vi "UI V7.1.1.vi"() -> ()   [LabVIEW 2017]
uses:
  <vilib>/Instr/_visa.llb/VISA Configure Serial Port (Instr).vi
  <vilib>/addons/Biomedical/Biosignal Measurements/Biosignal Preprocessing/Biosignal Rate Extractor (Waveform).vi
  <vilib>/addons/Biomedical/NI_BMTK_Measurements.lvlib
panel:
  out "?":bool
  out "?":bool
  out "CH1 PULSE Counter PM":u8
  out "CH2 PULSE Counter PM":i32
  out "CH1 PM":u8
  out "CH2 PM":dbl format="%#.6g"
  out "CH2":waveform(dbl)(graph)
  in  "stop":bool
  out "CH1":waveform(dbl)(graph)
  in  "Arduino Port":refnum<visa-resource-name>
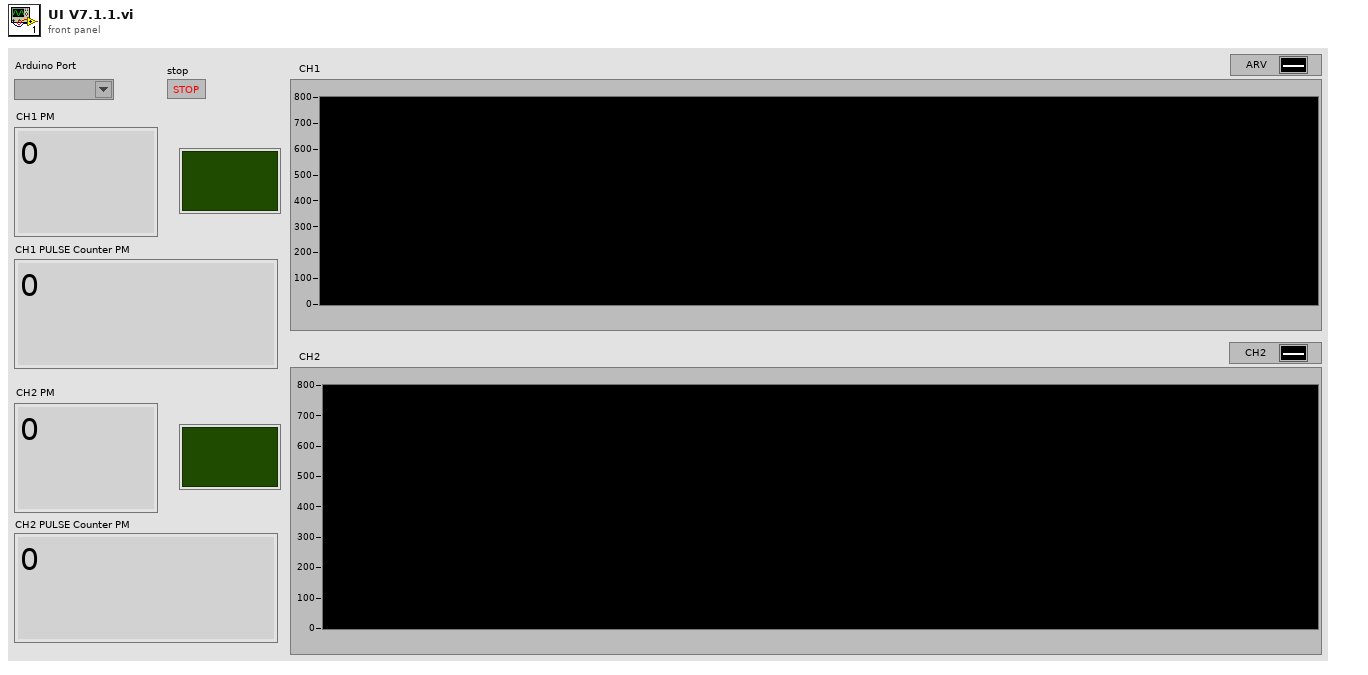
[diagram p1: front panel]
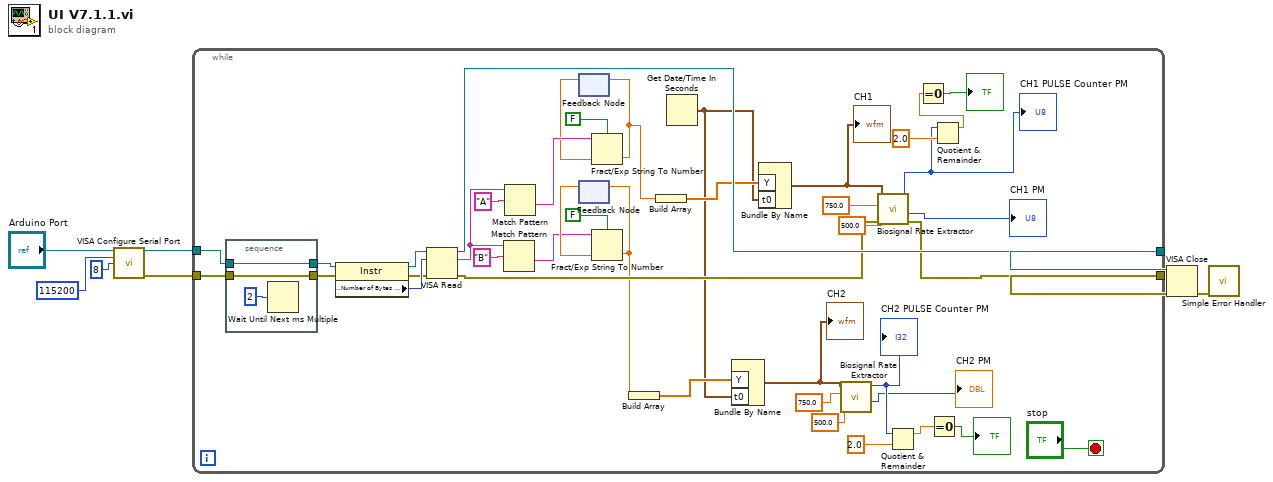
[diagram p0: block diagram]
diagram:
  n1 = call-poly "VISA Configure Serial Port"("VISA resource name"="Arduino Port", "baud rate (9600)"=u32 115200, "data bits (8)"=u16 8) -> ("VISA resource name out"=w5:refnum<visa-resource-name>, "error out"=w4:errorcluster)  [unwired: 11 in]
  n2 = while {
    tunnel: w5 -> [w49]
    tunnel: w4 -> [w47]
    tunnel: [w34] -> w3
    tunnel: [w28] -> w2
    stop <- "stop" stop-if-true
    n3 = stacked-sequence {
      tunnel: w49 -> [w52]
      tunnel: [w52] -> w48
      tunnel: w47 -> [w51]
      tunnel: [w51] -> w46
      frame #0 {
        n4 = Wait Until Next ms Multiple(millisecond multiple=u32 2) -> ()  [unwired: 1 out]
      }
    }
    n5 = property class="Instr"(reference=w48, error in=w46) -> (reference out=w45:refnum<visa-resource-name>, error out=w43:errorcluster, "Serial Settings:Number of Bytes at Serial Port"=w44:u32)
    n6 = VISA Read(VISA resource name=w45, byte count=w44, error in (no error)=w43) -> (VISA resource name out=w34:refnum<visa-resource-name>, read buffer=w33:string, error out=w29:errorcluster)  [unwired: 1 out]
    n7 = Match Pattern(string=w33, regular expression="B") -> (after substring=w32:string)  [unwired: 1 in, 3 out]
    n8 = Match Pattern(string=w33, regular expression="A") -> (after substring=w39:string)  [unwired: 1 in, 3 out]
    n9 = feedback #1() -> (w36:dbl)  [unwired: 1 in]
    n10 = feedback #2() -> (w35:dbl)  [unwired: 1 in]
    n11 = Fract/Exp String To Number(use system decimal point (T)=FALSE, string=w39, default (0 dbl)=w36) -> (number=w31:dbl)  [unwired: 1 in, 1 out]
    n12 = feedback-in #1(w31) -> ()
    n13 = Fract/Exp String To Number(use system decimal point (T)=FALSE, string=w32, default (0 dbl)=w35) -> (number=w21:dbl)  [unwired: 1 in, 1 out]
    n14 = feedback-in #2(w21) -> ()
    n15 = Build Array(w21) -> (w22:dbl[])
    n16 = Build Array(w31) -> (w30:dbl[])
    n17 = Get Date/Time In Seconds() -> (seconds since 1Jan1904=w13:timestamp)
    n18 = Bundle By Name("Y"=w22, "t0"=w13) -> (w23:waveform(dbl))  [unwired: 1 in]
    "CH2" <- w23
    n19 = Bundle By Name("Y"=w30, "t0"=w13) -> (w11:waveform(dbl))  [unwired: 1 in]
    "CH1" <- w11
    n20 = call-poly <vilib>:"Biosignal Rate Extractor.vi"("low threshold"=500.0, "high threshold"=750.0, "biosignal"=w23) -> ("number of cycles per minuets"=→"CH2 PM":i32, "number of cycles"=w16:i32)  [unwired: 5 in, 2 out]
    "CH2 PULSE Counter PM" <- w16
    n21 = call-poly <vilib>:"Biosignal Rate Extractor.vi"("error in (no error)"=w29, "low threshold"=500.0, "high threshold"=750.0, "biosignal"=w11) -> ("error out"=w28:errorcluster, "number of cycles per minuets"=→"CH1 PM":i32, "number of cycles"=w12:i32)  [unwired: 4 in, 1 out]
    "CH1 PULSE Counter PM" <- w12
    n22 = Quotient & Remainder(x=w16, y=2.0) -> (x-y*floor(x/y)=w17:dbl)  [unwired: 1 out]
    n23 = Equal To 0?(x=w17) -> (x = 0?=→"?":bool)
    n24 = Quotient & Remainder(x=w12, y=2.0) -> (x-y*floor(x/y)=w14:dbl)  [unwired: 1 out]
    n25 = Equal To 0?(x=w14) -> (x = 0?=→"?":bool)
  }
  n26 = VISA Close(VISA resource name=w3, error in (no error)=w2) -> (error out=w1:errorcluster)
  n27 = call <vilib>:"Simple Error Handler.vi"("error in (no error)"=w1) -> ()  [unwired: 4 in, 5 out]
